vi "Process Standard Output.vi"(8 "error in (no error)":errorcluster, 11 "VLC Wrapper in":refnum<class "VLC Wrapper.lvclass">) -> (0 "error out":errorcluster, 2 "Command output":string, 3 "VLC Wrapper out":refnum<class "VLC Wrapper.lvclass">)   [LabVIEW 2020, in "VLC Wrapper.lvclass"]
doc: "Process the response for a specific command. Child classes may override this method to process what is returned. The default behavior is to display the whole command response in a dialog box."
uses:
  VLC Wrapper.lvclass
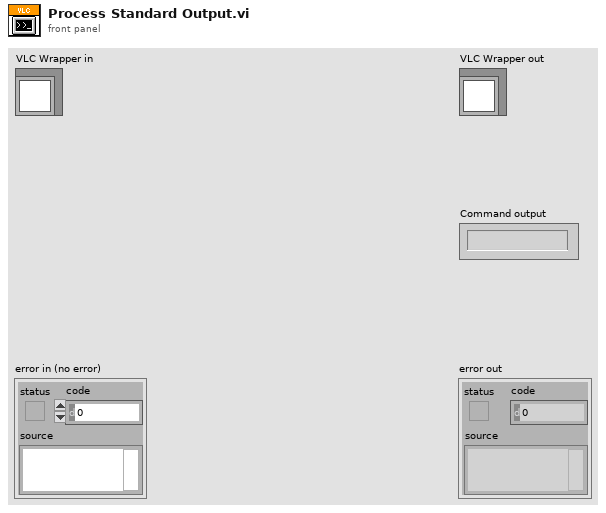
[diagram p1: front panel]
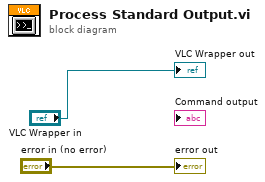
[diagram p0: block diagram]
diagram:
  "error out" <- "error in (no error)"
  "VLC Wrapper out" <- "VLC Wrapper in"
